vi "IMUread.vi"(11 "Channel Name":tag="B/I2C") -> (1 "Gyro":i16[](array[numeric]), 3 "Acc":i16[](array[numeric]))   [LabVIEW 2019]
doc: "The myRIO Project template acquires acceleration data from the onboard accelerometer and displays the changes of acceleration values in a waveform chart."
uses:
  <vilib>/myRIO/Instrument Drivers/Onboard IO/I2C/typedefs/I2C User Configuration.ctl
  <vilib>/myRIO/Instrument Drivers/Onboard IO/I2C/typedefs/I2C Transfer Rate.ctl
  <vilib>/Platform/TimedLoop/XDataNode/timing_clust.ctl
  <vilib>/Platform/TimedLoop/XDataNode/nitl_modes.ctl
  <vilib>/Platform/TimedLoop/XDataNode/wakeup.ctl
  <vilib>/myRIO/Common/Instrument Driver Framework/myRIO v1.0/UART/vis/myRIO v1.0 Close UART.vi
  <vilib>/Utility/error.llb/Error Cluster From Error Code.vi
  <vilib>/myRIO/Common/Instrument Driver Framework/myRIO v1.0/I2C/vis/myRIO v1.0 Configure I2C.vi
  <vilib>/myRIO/Common/Instrument Driver Framework/myRIO v1.0/I2C/vis/myRIO v1.0 Write I2C.vi
  <vilib>/myRIO/Common/Instrument Driver Framework/myRIO v1.0/I2C/vis/myRIO v1.0 Read I2C.vi
  <vilib>/myRIO/Common/Instrument Driver Framework/Utilities/vis/FPGA Ref Manager.vi
  <vilib>/myRIO/Common/Instrument Driver Framework/myRIO v1.0/myRIO v1.0 Reset FPGA.vi
  <vilib>/myRIO/Common/Instrument Driver Framework/myRIO v1.0/IRQ/vis/myRIO v1.0 IRQ Info FGV.vi
  <vilib>/myRIO/Common/Instrument Driver Framework/myRIO v1.0/IRQ/vis/myRIO v1.0 Timer IRQ Info FGV.vi
  <vilib>/myRIO/Common/Instrument Driver Framework/myRIO v1.0/IRQ/vis/myRIO v1.0 ISR Agent.vi
  <vilib>/myRIO/Instrument Drivers/Utilities/vis/Reset Index.vi
  <vilib>/myRIO/Common/Instrument Driver Framework/myRIO v1.0/Resource Manager/vis/myRIO v1.0 Block Write Resource Manager.vi
  <vilib>/platform/TimedLoop/XDataNode/XDataNode.xnode
  <vilib>/myRIO/Instrument Drivers/Utilities/Utilities.lvlib
  <vilib>/myRIO/Instrument Drivers/Onboard IO/I2C/I2C.lvlib
  <vilib>/Platform/TimedLoop/XDataNode/XDNodeRunTimeDep.lvlib
panel:
  in  "Stop Button":bool
  out "Gyro Chart":cluster{dbl, dbl, dbl}(graph)
  out "Acc Chart":cluster{dbl, dbl, dbl}(graph)
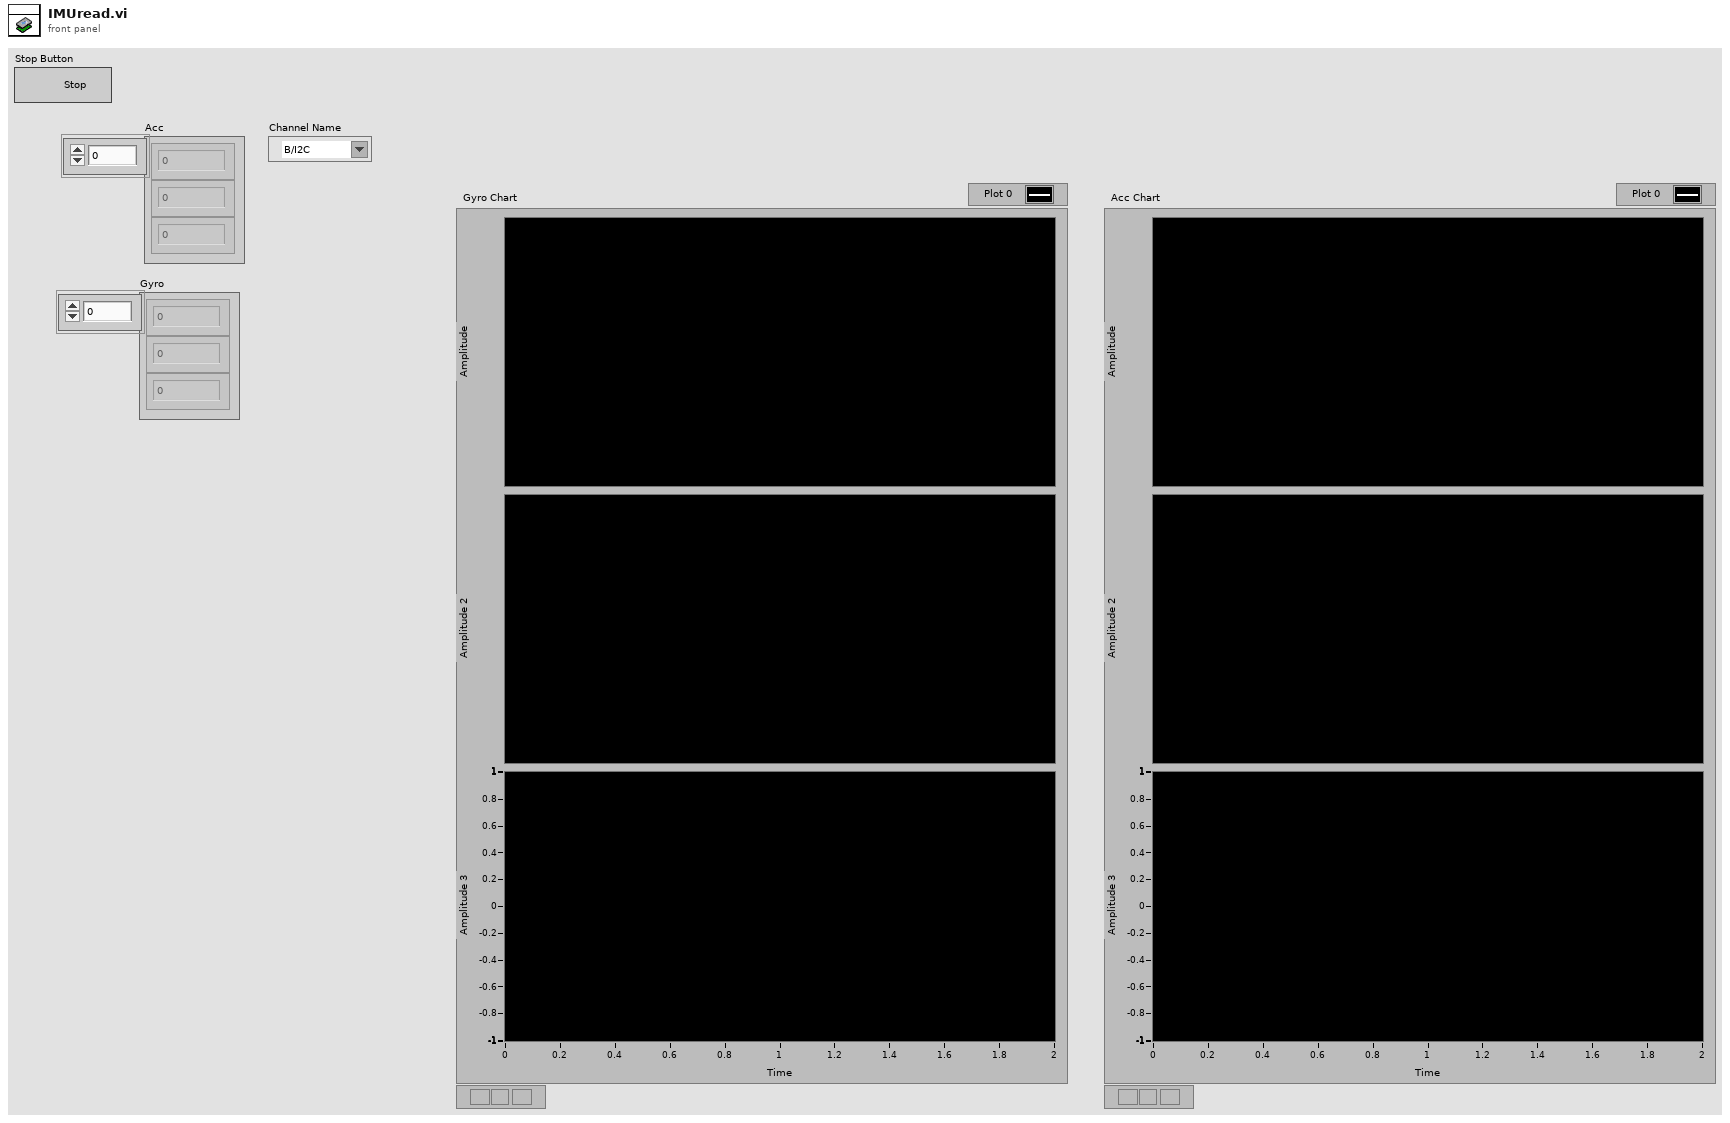
[diagram p1: front panel]
types:
  T1 = typedef "I2C.lvlib/I2C User Configuration.ctl" = cluster{"I2C Transfer Rate":T2}
  T2 = typedef "I2C.lvlib/I2C Transfer Rate.ctl" = enum16{"Standard mode (100 kbps)", "Fast mode (400 kbps)"}
  T3 = typedef "I2C.lvlib/I2C Reference.ctl" = cluster{"myRIO Reference":T4, "I2C Channels Enum":T8, "I2C Configuration":T9}
  T4 = typedef "myRIO Generic Hardware Reference.ctl" = cluster{"myRIO Model":T5, "myRIO Hardware Reference":T6}
  T5 = typedef "Hardware Version Enum.ctl" = enum16{"Unknown", "myRIO-1900", "myRIO-1950", "roboRIO", "NI ELVIS RIO CM", "ELVIS III"}
  T6 = typedef "myRIO v1.0 Reference.ctl" = cluster{"Generic FPGA Reference":T7, "Allow multiple opens":bool}
  T7 = typedef "Generic FPGA Reference.ctl" = refnum<k20>
  T8 = typedef "I2C Channels Enum.ctl" = enum16{"Not Connected", "A/I2C", "B/I2C", "I2C/I2C"}
  T9 = typedef "I2C.lvlib/I2C Configuration.ctl" = cluster{"I2C Transfer Rate":T2}
  T10 = typedef "XDNodeRunTimeDep.lvlib/timing_clust.ctl" = cluster{"Expected End [f-1]":u64, "Actual End [f-1]":u64, "Finished Late? [f-1]":bool, "Expected End [i-1]":u64, "Actual End [i-1]":u64, "Finished Late? [i-1]":bool, "Expected Start [i]":u64, "Actual Start [i]":u64, "Expected Start [f]":u64, "Actual Start [f]":u64, "Source Name":string, "Structure Name":string, "Period":i64, "Deadline":i64, "Offset":i64, "Start":i64, "Priority":i32, "Timeout":i32, "Mode":T11, "Wakeup Reason":T12, "Error":errorcluster, "Source Type":string, "Secondary Source Type":string, "Global End Time":u64, "Global Start Time":u64, "Frame Duration":u64, "Iteration Duration":u64, "Assigned CPU":i32, "I/O Scan Engine Mode":u32}
  T11 = typedef "XDNodeRunTimeDep.lvlib/nitl_modes.ctl" = enum32{"No Change", "Process missed periods, maintain original phase", "Discard missed periods, maintain original phase", "Process missed periods, ignore original phase", "Discard missed periods, ignore original phase"}
  T12 = typedef "XDNodeRunTimeDep.lvlib/wakeup.ctl" = enum32{"Normal", "Aborted", "Asynchronous wakeup", "Timing source error", "Timed loop error", "Timeout"}
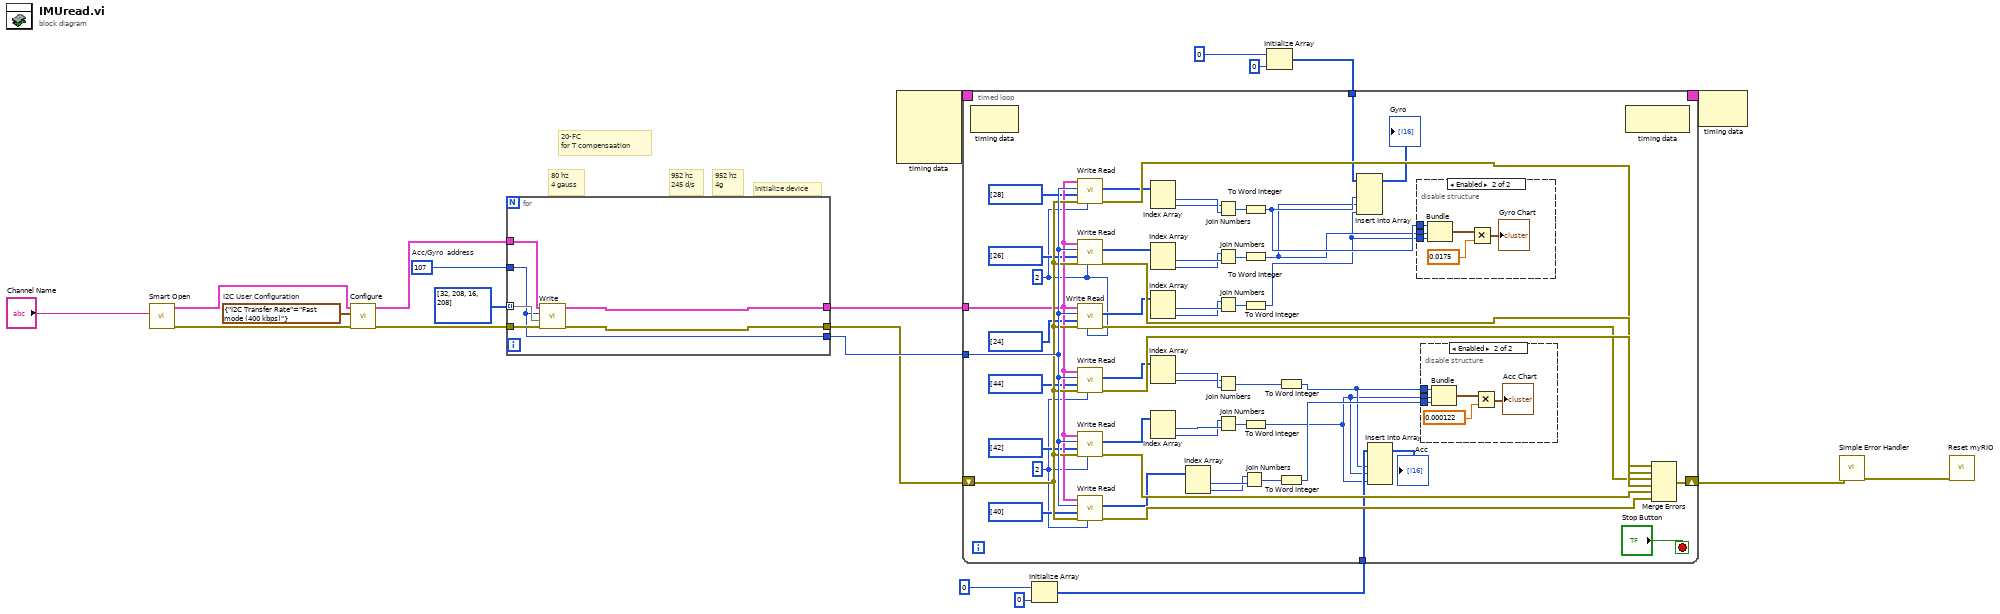
[diagram p0: block diagram]
diagram:
  w17 = u8 107  # Acc/Gyro  address
  w20 = T1 {"I2C Transfer Rate"=enum."Fast mode (400 kbps)"}  # I2C User Configuration
  # "20-FC\nfor T compensaation"
  # "80 hz\n4 gauss"
  # "952 hz\n4g"
  # "952 hz\n245 d/s"
  # "Initialize device"
  n1 = call <vilib>:"Smart Open.vi"("Channel Name"="Channel Name") -> ("error out"=w18:errorcluster, "I2C Ref Out"=w19:T3)  [unwired: 9 in]
  n2 = call <vilib>:"Configure.vi"("error in (no error)"=w18, "I2C User Configuration"=w20, "I2C Ref In"=w19) -> ("error out"=w13:errorcluster, "I2C Ref Out"=w14:T3)  [unwired: 7 in]
  n3 = for {
    tunnel: [w22] -> w12
    tunnel: [w23] -> w11
    tunnel: [w24] -> w15
    tunnel: u8[][] [[32, 208], [16, 208]] ("Bytes to Write") -> [w25] mode=indexing
    tunnel: w14 -> [w27]
    tunnel: w13 -> [w26]
    tunnel: w17 -> [w24]
    n4 = call <vilib>:"Write.vi"("error in (no error)"=w26, "Bytes to Write"=w25, "Slave Address (7-bit)"=w24, "I2C Ref In"=w27) -> ("error out"=w22:errorcluster, "I2C Ref Out"=w23:T3)  [unwired: 6 in]
  }
  n5 = node-c288() -> (w2:T10)  [unwired: 4 in]
  n6 = Initialize Array(i16 0 ("element"), 0 ("dimension size")) -> (w6:i16[])
  n7 = Initialize Array(i16 0 ("element"), 0 ("dimension size")) -> (w3:i16[])
  n8 = timed-loop {
    timing: w2 -> [_]
    timing-out: [_] -> w1
    tunnel: w15 -> [w77]
    tunnel: w11 -> [w72]
    tunnel: w6 -> [w70]
    tunnel: w3 -> [w69]
    shift-right: [w71] -> w10
    shift-left: w12 -> [w73]
    stop <- "Stop Button" stop-if-true
    w37 = u32 2 ("Byte Count")
    w53 = u32 2 ("Byte Count")
    n9 = node-c288() -> ()  [unwired: 1 in, 1 out]
    n10 = call <vilib>:"Write Read.vi"("Byte Count"=w37, "error in (no error)"=w73, "Bytes to Write"=u8[] [28], "Slave Address (7-bit)"=w77, "I2C Ref In"=w72) -> ("error out"=w74:errorcluster, "Bytes Read"=w45:u8[])  [unwired: 3 in, 1 out]
    n11 = call <vilib>:"Write Read.vi"("Byte Count"=w37, "error in (no error)"=w73, "Bytes to Write"=u8[] [26], "Slave Address (7-bit)"=w77, "I2C Ref In"=w72) -> ("error out"=w75:errorcluster, "Bytes Read"=w47:u8[])  [unwired: 3 in, 1 out]
    n12 = call <vilib>:"Write Read.vi"("Byte Count"=w37, "error in (no error)"=w73, "Bytes to Write"=u8[] [24], "Slave Address (7-bit)"=w77, "I2C Ref In"=w72) -> ("error out"=w76:errorcluster, "Bytes Read"=w49:u8[])  [unwired: 3 in, 1 out]
    n13 = call <vilib>:"Write Read.vi"("Byte Count"=w53, "error in (no error)"=w73, "Bytes to Write"=u8[] [44], "Slave Address (7-bit)"=w77, "I2C Ref In"=w72) -> ("error out"=w80:errorcluster, "Bytes Read"=w61:u8[])  [unwired: 3 in, 1 out]
    n14 = call <vilib>:"Write Read.vi"("Byte Count"=w53, "error in (no error)"=w73, "Bytes to Write"=u8[] [42], "Slave Address (7-bit)"=w77, "I2C Ref In"=w72) -> ("error out"=w79:errorcluster, "Bytes Read"=w63:u8[])  [unwired: 3 in, 1 out]
    n15 = call <vilib>:"Write Read.vi"("Byte Count"=w53, "error in (no error)"=w73, "Bytes to Write"=u8[] [40], "Slave Address (7-bit)"=w77, "I2C Ref In"=w72) -> ("error out"=w78:errorcluster, "Bytes Read"=w65:u8[])  [unwired: 3 in, 1 out]
    n16 = Index Array "Index Array"(array=w45) -> (element #1=w43:u8, element #2=w42:u8)  [unwired: 2 in]
    n17 = Index Array "Index Array"(array=w47) -> (element #1=w41:u8, element #2=w40:u8)  [unwired: 2 in]
    n18 = Index Array "Index Array"(array=w49) -> (element #1=w39:u8, element #2=w38:u8)  [unwired: 2 in]
    n19 = Index Array "Index Array"(array=w61) -> (element #1=w59:u8, element #2=w58:u8)  [unwired: 2 in]
    n20 = Index Array "Index Array"(array=w63) -> (element #1=w57:u8, element #2=w56:u8)  [unwired: 2 in]
    n21 = Index Array "Index Array"(array=w65) -> (element #1=w55:u8, element #2=w54:u8)  [unwired: 2 in]
    n22 = Join Numbers(hi=w42, lo=w43) -> ((hi.lo)=w52:u16)
    n23 = Join Numbers(hi=w40, lo=w41) -> ((hi.lo)=w51:u16)
    n24 = Join Numbers(hi=w38, lo=w39) -> ((hi.lo)=w50:u16)
    n25 = Join Numbers(hi=w58, lo=w59) -> ((hi.lo)=w68:u16)
    n26 = Join Numbers(hi=w56, lo=w57) -> ((hi.lo)=w67:u16)
    n27 = Join Numbers(hi=w54, lo=w55) -> ((hi.lo)=w66:u16)
    n28 = To Word Integer(number=w52) -> (16bit integer=w32:i16)
    n29 = To Word Integer(number=w51) -> (16bit integer=w31:i16)
    n30 = To Word Integer(number=w50) -> (16bit integer=w30:i16)
    n31 = To Word Integer(number=w67) -> (16bit integer=w34:i16)
    n32 = To Word Integer(number=w68) -> (16bit integer=w35:i16)
    n33 = To Word Integer(number=w66) -> (16bit integer=w36:i16)
    n34 = Insert Into Array(array=w69, new element #1=w32, new element #2=w31, new element #3=w30) -> (→"Gyro":i16[])  [unwired: 1 in]
    n35 = Insert Into Array(array=w70, new element #1=w35, new element #2=w34, new element #3=w34) -> (→"Acc":i16[])  [unwired: 1 in]
    n36 = disable-structure shown="Enabled" {
      disable-tunnel: w32 -> [_ w84]
      disable-tunnel: w31 -> [_ w83]
      disable-tunnel: w30 -> [_ w82]
      frame Disabled {
      }
      frame Enabled {
        n37 = Bundle "Bundle"(w84, w83, w82) -> (w86:cluster{i16, i16, i16})  [unwired: 1 in]
        n38 = Multiply(x=w86, y=0.0175) -> (x*y=→"Gyro Chart":cluster{dbl, dbl, dbl})
      }
    }
    n39 = disable-structure shown="Enabled" {
      disable-tunnel: w35 -> [_ w89]
      disable-tunnel: w34 -> [_ w88]
      disable-tunnel: w36 -> [_ w87]
      frame Disabled {
      }
      frame Enabled {
        n40 = Bundle "Bundle"(w89, w88, w87) -> (w91:cluster{i16, i16, i16})  [unwired: 1 in]
        n41 = Multiply(x=w91, y=0.000122) -> (x*y=→"Acc Chart":cluster{dbl, dbl, dbl})
      }
    }
    n42 = node-c288() -> ()  [unwired: 1 in, 1 out]
    n43 = Merge Errors(w74, w75, w76, w80, w79, w78) -> (w71:errorcluster)
  }
  n44 = node-c288(w1) -> ()  [unwired: 1 out]
  n45 = call <vilib>:"Simple Error Handler.vi"("error in (no error)"=w10) -> ("error out"=w21:errorcluster)  [unwired: 4 in, 4 out]
  n46 = call <vilib>:"Reset myRIO.vi"("error in (no error)"=w21) -> ()  [unwired: 10 in, 1 out]
